vi "IntegerToBoolean.vi"(11 "Integer input":i32) -> (3 "Boolean":bool=TRUE)   [LabVIEW 2020]
uses:
  <vilib>/Utility/error.llb/Error Cluster From Error Code.vi
  <vilib>/ErrorRing/Error Ring.xnode
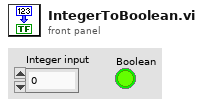
[diagram p1: front panel]
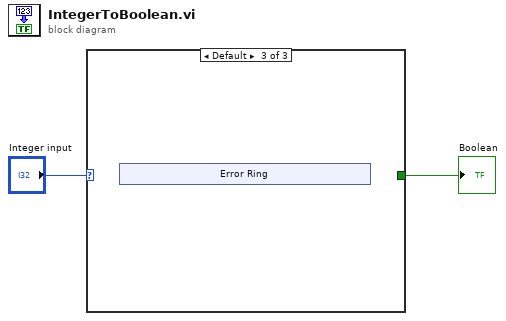
[diagram p0: block diagram]
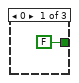
[diagram p2: hidden frame]
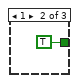
[diagram p3: hidden frame]
diagram:
  n1 = case shown="Default" "Integer input" {
    tunnel: [FALSE TRUE _] -> w1
    frame 0 {
    }
    frame 1 {
    }
    frame Default {
      n2 = xnode "Error Ring"() -> ()  [unwired: 1 out]
    }
  }
  "Boolean" <- w1
